vi "Measure.vi"(8 "error in":errorcluster, 11 "4322 in":refnum<class "4322.lvclass">) -> (0 "error out":errorcluster, 3 "4322 out":refnum<class "4322.lvclass">)   [LabVIEW 2019, in "4322.lvlib" / "4322.lvclass"]
uses:
  Library/4322.lvclass
  builds/Instruments/Analog-Output.lvlibp/Library/Analog-Output.lvclass
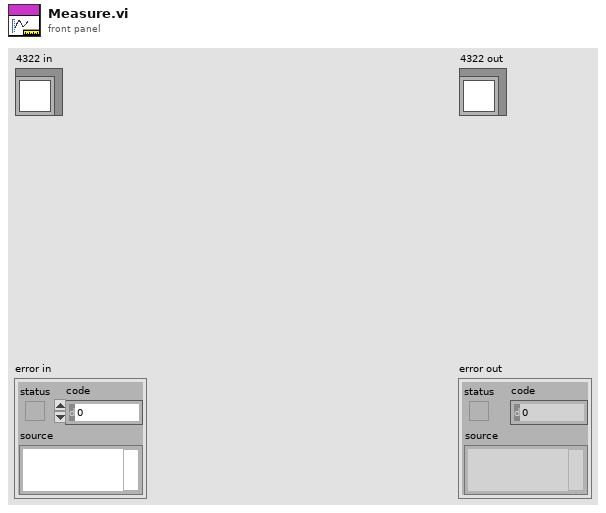
[diagram p1: front panel]
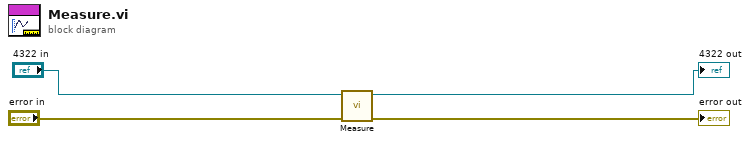
[diagram p0: block diagram]
diagram:
  n1 = call-parent "Measure.vi"("error in"="error in", "Analog-Output in"="4322 in") -> ("error out"=→"error out":errorcluster, "Analog-Output out"=→"4322 out":refnum<class "4322.lvclass">)  [unwired: 8 in]
